vi "niRFUtil WFM Detect Edge.vi"   [LabVIEW 2015, in "niRFUtil.lvlib"]
uses:
  niRFUtil.lvlib
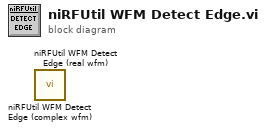
[diagram p0: block diagram]
diagram:
  n1 = call "niRFUtil WFM Detect Edge (complex wfm).vi"() -> ()  [unwired: 12 in, 4 out]
  n2 = call "niRFUtil WFM Detect Edge (real wfm).vi"() -> ()  [unwired: 12 in, 4 out]
